vi "CRC_Calculator.vi"() -> ()   [LabVIEW 2019]
panel:
  in  "Init":u16 format="%x"
  in  "Poly":u16=33800 format="%x"
  out "lo(x)":u8 format="%x"
  out "hi(x)":u8 format="%x"
  in  "Binário APP":path
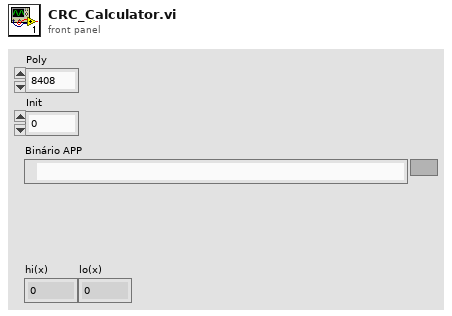
[diagram p1: front panel]
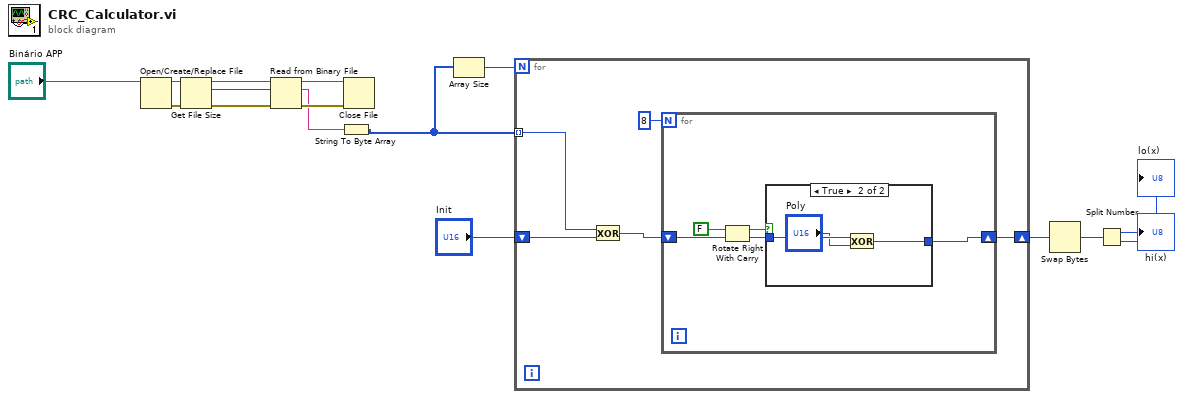
[diagram p0: block diagram]
diagram:
  n1 = Open/Create/Replace File(file path (use dialog)="Binário APP") -> (refnum out=w7:refnum<file>, error out=w8:errorcluster)  [unwired: 5 in, 1 out]
  n2 = Get File Size(file=w7, error in=w8) -> (refnum out=w9:refnum<file>, size (in bytes)=w3:i64, 0:w10:errorcluster)
  n3 = Read from Binary File(8:w10, 10:w3, 11:w9) -> (0:w11:errorcluster, 2:w6:string, 3:w12:refnum<file>)  [unwired: 3 in, 1 out]
  n4 = String To Byte Array(string=w6) -> (unsigned byte array=w4:u8[])
  n5 = Close File(refnum=w12, error in=w11) -> ()  [unwired: 2 out]
  n6 = Array Size(array=w4) -> (size(s)=w15:i32)
  n7 = for {
    N: w15 -> [_]
    tunnel: w4 -> [w17] mode=indexing
    shift-right: [w20] -> w14
    shift-left: "Init" -> [w19]
    n8 = Exclusive Or(1:w19, 2:w17) -> (0:w21:u16)
    n9 = for {
      N: 8 -> [_]
      shift-right: [w22] -> w20
      shift-left: w21 -> [w26]
      n10 = Rotate Right With Carry(2:w26, 3:FALSE ("carry")) -> (0:w23:u16, 1:w24:bool)
      n11 = case shown="True" w24 {
        tunnel: w23 -> [w27 w30]
        tunnel: [w27 w28] -> w22
        frame False {
        }
        frame True {
          n12 = Exclusive Or(1:"Poly", 2:w30) -> (0:w28:u16)
        }
      }
    }
  }
  n13 = Swap Bytes(anything=w14) -> (byte swapped=w13:u16)
  n14 = Split Number(x=w13) -> (hi(x)=→"hi(x)":u8, lo(x)=→"lo(x)":u8)
